vi "Generate Concrete Relative Paths File.vi"() -> ()   [LabVIEW 2023, in "Concrete Classes.lvlib"]
uses:
  Concrete Classes.lvlib
  Test Caller Actor/Abstract Class/Abstract Class.lvclass
  Class 1/Class 1.lvclass
  C:/Projects/Shared Libraries/Class Loader/Test Caller Actor/Abstract Class/Abstract Class.lvclass
  Class 2/Class 2.lvclass
  Class 3/Class 3 Folder/Class 3.lvclass
  Class 4/Class 4.lvclass
  Class 5/Class 5.lvclass
  Class 6/Class 6.lvclass
  Class 7/Class 7.lvclass
  Class 8/Class 8.lvclass
  Class 9/Class 9.lvclass
  Class 10/Class 10.lvclass
  Class Loader/Class Loader/Class Loader.lvclass
panel:
  out "error out":errorcluster
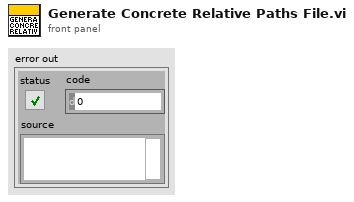
[diagram p1: front panel]
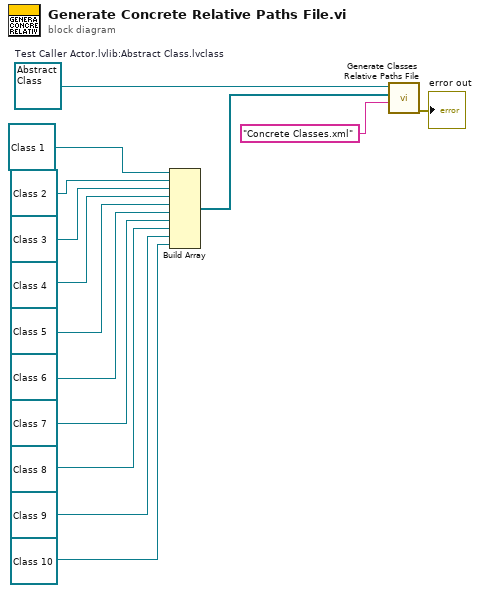
[diagram p0: block diagram]
diagram:
  w14 = refnum<class "Abstract Class.lvclass"> refnum  # Test Caller Actor.lvlib:Abstract Class.lvclass
  n1 = Build Array(refnum<class "Class 1.lvclass"> refnum ("Concrete Classes.lvlib:Class 1.lvclass"), refnum<class "Class 2.lvclass"> refnum ("Concrete Classes.lvlib:Class 2.lvclass"), refnum<class "Class 3.lvclass"> refnum ("Concrete Classes.lvlib:Class 3.lvclass"), refnum<class "Class 4.lvclass"> refnum ("Concrete Classes.lvlib:Class 4.lvclass"), refnum<class "Class 5.lvclass"> refnum ("Concrete Classes.lvlib:Class 5.lvclass"), refnum<class "Class 6.lvclass"> refnum ("Concrete Classes.lvlib:Class 6.lvclass"), refnum<class "Class 7.lvclass"> refnum ("Concrete Classes.lvlib:Class 7.lvclass"), refnum<class "Class 8.lvclass"> refnum ("Concrete Classes.lvlib:Class 8.lvclass"), refnum<class "Class 9.lvclass"> refnum ("Concrete Classes.lvlib:Class 9.lvclass"), refnum<class "Class 10.lvclass"> refnum ("Concrete Classes.lvlib:Class 10.lvclass")) -> (w3:refnum<class "Abstract Class.lvclass">[])
  n2 = call "Generate Classes Relative Paths File.vi"("Relative Paths File Name"="Concrete Classes.xml", "Classes"=w3, "Reference Class"=w14) -> ("error out"=→"error out":errorcluster)  [unwired: 8 in]
